vi "wheel_turn.vi"(8 "에러 입력":errorcluster, 10 "wanted angle(deg)":dbl, 11 "FPGA VI 참조 입력":refnum<k20>) -> (0 "에러 출력":errorcluster, 3 "FPGA VI 참조 출력":refnum<k20>)   [LabVIEW 2019]
uses:
  <vilib>/Platform/TimedLoop/XDataNode/timing_clust.ctl
  <vilib>/Platform/TimedLoop/XDataNode/nitl_modes.ctl
  <vilib>/Platform/TimedLoop/XDataNode/wakeup.ctl
  <vilib>/Utility/error.llb/Error Cluster From Error Code.vi
  <vilib>/rvi/errors/niLvFpgaAdjustHostInterfaceError.vi
  <vilib>/rvi/interface/nirviReadWriteControl/nirviReadWriteControl.xnode
  <vilib>/Platform/TimedLoop/XDataNode/XDataNode.xnode
  <vilib>/Platform/TimedLoop/XDataNode/XDNodeRunTimeDep.lvlib
  <vilib>/rvi/interface/Simulation/niFpgaSimulationCallBeginRW.vi
  NiFpgaLv.dll
panel:
  out "숫자형":dbl
  out "둘 다 돌았나?":bool
  in  "정지":bool
  out "mm/ms":dbl
  out "R_이동 거리":dbl
  out "R_Encoder":i32
  out "L_이동 거리":dbl
  out "L_encoder":i32
  out "타임아웃":i32
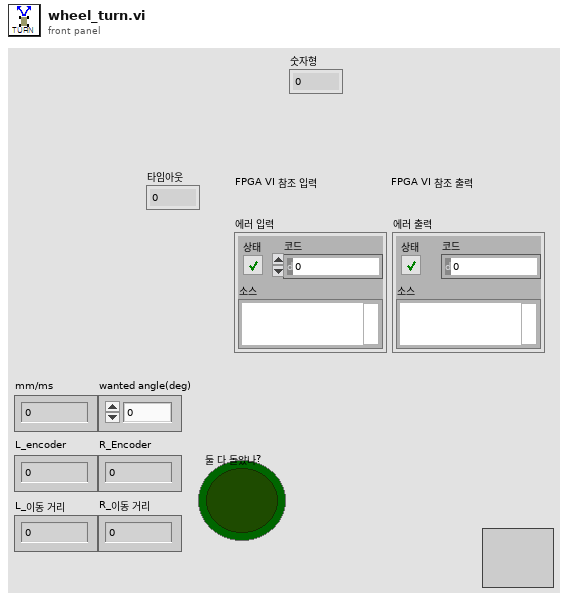
[diagram p1: front panel]
types:
  T1 = typedef "XDNodeRunTimeDep.lvlib/timing_clust.ctl" = cluster{"Expected End [f-1]":u64, "Actual End [f-1]":u64, "Finished Late? [f-1]":bool, "Expected End [i-1]":u64, "Actual End [i-1]":u64, "Finished Late? [i-1]":bool, "Expected Start [i]":u64, "Actual Start [i]":u64, "Expected Start [f]":u64, "Actual Start [f]":u64, "Source Name":string, "Structure Name":string, "Period":i64, "Deadline":i64, "Offset":i64, "Start":i64, "Priority":i32, "Timeout":i32, "Mode":T2, "Wakeup Reason":T3, "Error":errorcluster, "Source Type":string, "Secondary Source Type":string, "Global End Time":u64, "Global Start Time":u64, "Frame Duration":u64, "Iteration Duration":u64, "Assigned CPU":i32, "I/O Scan Engine Mode":u32}
  T2 = typedef "XDNodeRunTimeDep.lvlib/nitl_modes.ctl" = enum32{"No Change", "Process missed periods, maintain original phase", "Discard missed periods, maintain original phase", "Process missed periods, ignore original phase", "Discard missed periods, ignore original phase"}
  T3 = typedef "XDNodeRunTimeDep.lvlib/wakeup.ctl" = enum32{"Normal", "Aborted", "Asynchronous wakeup", "Timing source error", "Timed loop error", "Timeout"}
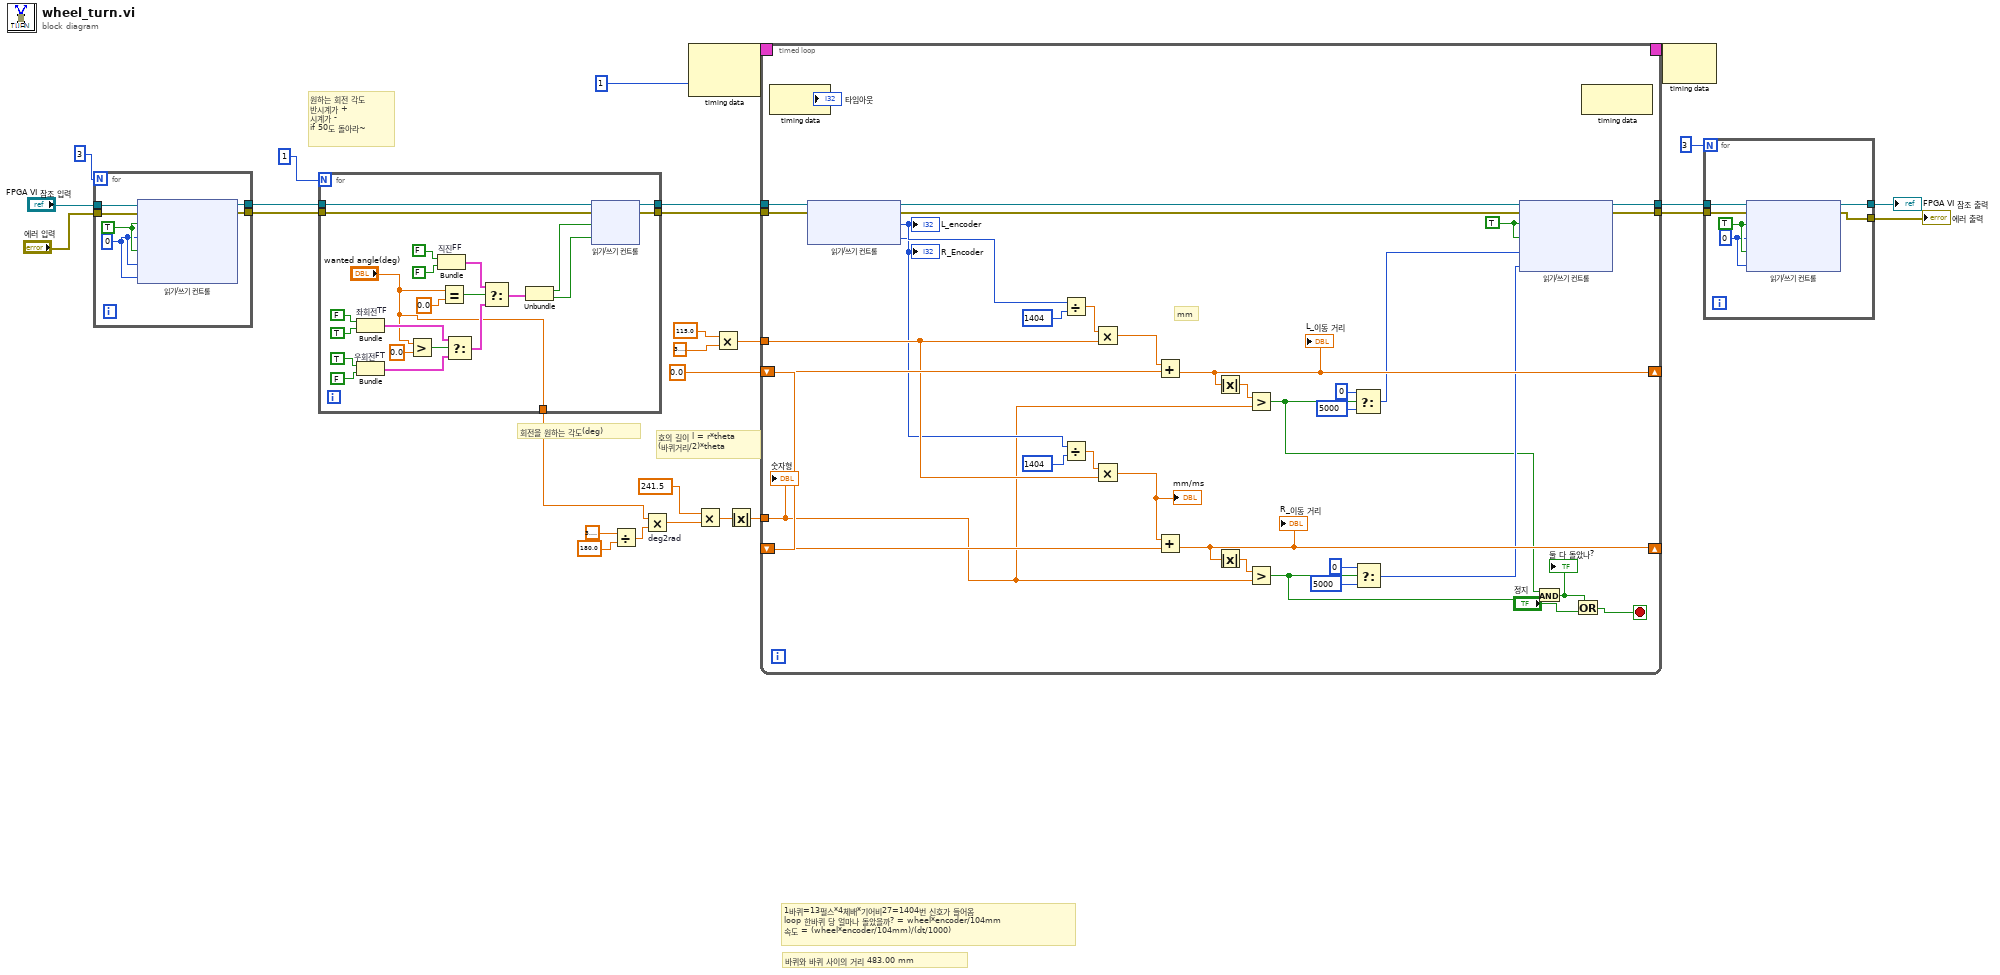
[diagram p0: block diagram]
diagram:
  w19 = 0.0
  # "원하는 회전 각도\n반시계가 +\n시계가 -\nif 50도 돌아라~"
  # "호의 길이 l = r*theta\n(바퀴거리/2)*theta"
  # "회전을 원하는 각도(deg)"
  # "바퀴와 바퀴 사이의 거리 483.00 mm"
  # "1바퀴=13펄스*4체배*기어비27=1404번 신호가 들어옴\nloop 한바퀴 당 얼마나 돌았을까? = wheel*encoder/104mm\n속도 = (wheel*encoder/104mm)/(dt/1000)"
  n1 = for {
    N: 3 -> [_]
    tunnel: [w34] -> w16
    tunnel: [w33] -> w15
    tunnel: "에러 입력" -> [w30]
    tunnel: "FPGA VI 참조 입력" -> [w29]
    w31 = 0 ("pwm input(escon)")
    w32 = TRUE ("encoder reset")
    n2 = xnode "읽기/쓰기 컨트롤"("FPGA VI 참조 입력"=w29, "에러 입력"=w30, "encoder reset"=w32, "pwm input"=w31, "R_encoder reset"=w32, "R_pwm input"=w31, "직동_pwm input"=w31) -> ("FPGA VI 참조 출력"=w34:refnum<k20>, "에러 출력"=w33:errorcluster)
  }
  n3 = for {
    N: 1 -> [_]
    tunnel: [w39] -> w18
    tunnel: [w38] -> w17
    tunnel: w16 -> [w37]
    tunnel: w15 -> [w36]
    tunnel: ["wanted angle(deg)"] -> w10
    n4 = Bundle "좌회전TF"(FALSE, TRUE) -> (w42:cluster{bool, bool})  [unwired: 1 in]
    n5 = Bundle "우회전FT"(TRUE, FALSE) -> (w41:cluster{bool, bool})  [unwired: 1 in]
    n6 = Greater?(x="wanted angle(deg)", y=0.0) -> (0:w44:bool)
    n7 = Bundle "직진FF"(FALSE, FALSE) -> (w48:cluster{bool, bool})  [unwired: 1 in]
    n8 = Equal?(x="wanted angle(deg)", y=0.0) -> (x = y?=w56:bool)
    n9 = Select(t=w42, s=w44, f=w41) -> (s? t:f=w40:cluster{bool, bool})
    n10 = Select(t=w48, s=w56, f=w40) -> (s? t:f=w47:cluster{bool, bool})
    n11 = Unbundle(w47) -> (w46:bool, w45:bool)
    n12 = xnode "읽기/쓰기 컨트롤"("FPGA VI 참조 입력"=w37, "에러 입력"=w36, "L_dir"=w46, "R_dir"=w45) -> ("FPGA VI 참조 출력"=w39:refnum<k20>, "에러 출력"=w38:errorcluster)
  }
  n13 = Divide(x=3.141592653589793, y=180.0) -> (x/y=w11:dbl)
  n14 = Multiply "deg2rad"(x=w10, y=w11) -> (x*y=w8:dbl)
  n15 = node-c288(i64 1 ("주기")) -> (w28:T1)  [unwired: 1 in]
  n16 = Multiply(x=241.5, y=w8) -> (x*y=w2:dbl)
  n17 = Multiply(x=115.0, y=3.141592653589793) -> (x*y=w21:dbl)
  n18 = Absolute Value(x=w2) -> (abs(x)=w1:dbl)
  n19 = timed-loop {
    timing: w28 -> [_]
    timing-out: [_] -> w27
    tunnel: [w90] -> w26
    tunnel: [w89] -> w25
    tunnel: w21 -> [w83]
    shift-right: [w87] -> _
    shift-left: w19 -> [w84]
    shift-right: [w86] -> _
    shift-left: w19 -> [w85]
    tunnel: w18 -> [w80]
    tunnel: w17 -> [w79]
    tunnel: w1 -> [w78]
    stop <- w57 stop-if-true
    w88 = TRUE ("encoder reset")
    # "mm"
    n20 = node-c288() -> (→"타임아웃":i32)  [unwired: 1 in]
    n21 = xnode "읽기/쓰기 컨트롤"("FPGA VI 참조 입력"=w80, "에러 입력"=w79) -> ("FPGA VI 참조 출력"=w59:refnum<k20>, "에러 출력"=w58:errorcluster, "Encoder  (4x)"=w82:i32, "R_Encoder  (4x)"=w81:i32)
    "L_encoder" <- w82
    "R_Encoder" <- w81
    n22 = Divide(x=w82, y=1404) -> (x/y=w76:dbl)
    n23 = Divide(x=w81, y=1404) -> (x/y=w72:dbl)
    n24 = Multiply(x=w76, y=w83) -> (x*y=w70:dbl)
    n25 = Multiply(x=w72, y=w83) -> (x*y=w73:dbl)
    "mm/ms" <- w73
    n26 = Add(x=w70, y=w84) -> (x+y=w87:dbl)
    "L_이동 거리" <- w87
    n27 = Add(x=w73, y=w85) -> (x+y=w86:dbl)
    "R_이동 거리" <- w86
    n28 = Absolute Value(x=w87) -> (abs(x)=w75:dbl)
    n29 = Absolute Value(x=w86) -> (abs(x)=w71:dbl)
    n30 = Greater?(x=w75, y=w78) -> (0:w62:bool)
    n31 = Greater?(x=w71, y=w78) -> (0:w63:bool)
    n32 = Select(t=0, s=w62, f=5000) -> (s? t:f=w64:i32)
    n33 = Select(t=0, s=w63, f=5000) -> (s? t:f=w67:i32)
    n34 = xnode "읽기/쓰기 컨트롤"("FPGA VI 참조 입력"=w59, "에러 입력"=w58, "encoder reset"=w88, "R_encoder reset"=w88, "pwm input"=w64, "R_pwm input"=w67) -> ("FPGA VI 참조 출력"=w90:refnum<k20>, "에러 출력"=w89:errorcluster)
    n35 = And(x=w62, y=w63) -> (x .and. y?=w61:bool)
    "둘 다 돌았나?" <- w61
    n36 = Or(x=w61, y="정지") -> (x .or. y?=w57:bool)
    n37 = node-c288() -> ()  [unwired: 1 in, 1 out]
    "숫자형" <- w78
  }
  n38 = node-c288(w27) -> ()  [unwired: 1 out]
  n39 = for {
    N: 3 -> [_]
    tunnel: w26 -> [w100]
    tunnel: w25 -> [w99]
    tunnel: [w96] -> w4
    tunnel: [w95] -> w3
    w97 = 0 ("pwm input(escon)")
    w98 = TRUE ("encoder reset")
    n40 = xnode "읽기/쓰기 컨트롤"("FPGA VI 참조 입력"=w100, "에러 입력"=w99, "encoder reset"=w98, "pwm input"=w97, "R_encoder reset"=w98, "R_pwm input"=w97) -> ("FPGA VI 참조 출력"=w95:refnum<k20>, "에러 출력"=w96:errorcluster)
  }
  "FPGA VI 참조 출력" <- w3
  "에러 출력" <- w4
